vi "Restart_OGI_COMS.vi"   [LabVIEW 2011]
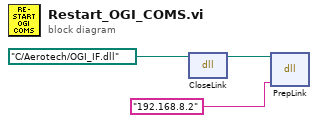
[diagram p0: block diagram]
diagram:
  n1 = dll-call lib="C:/Aerotech/Drivers/OGI_IF.dll" fn="CloseLink"(path in=path "C:/Aerotech/OGI_IF.dll") -> (path out=w1:path)  [unwired: 2 in, 2 out]
  n2 = dll-call lib="C:/Aerotech/Drivers/OGI_IF.dll" fn="PrepLink"(path in=w1, "IPAddress"="192.168.8.2") -> ()  [unwired: 2 in, 4 out]
